vi "Build Rearange Frames by Index Array.vi"(9 "New Position":i32, 10 "Current Position":i32, 11 "N":i32) -> (2 "New Positions Array":i32[](array[numeric]))   [LabVIEW 2020]
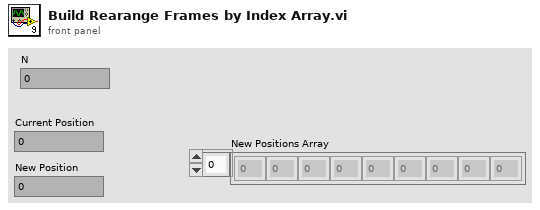
[diagram p1: front panel]
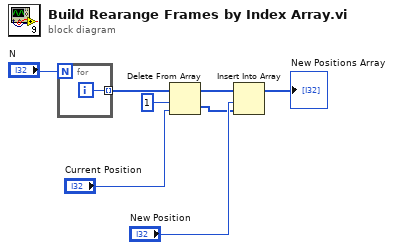
[diagram p0: block diagram]
diagram:
  n1 = for {
    N: "N" -> [_]
    tunnel: [w9] -> w4 mode=indexing
    i -> [w9]
  }
  n2 = Delete From Array(array=w4, length=1, index="Current Position") -> (deleted portion=w2:i32[], array with subset deleted=w1:i32[])
  n3 = Insert Into Array(array=w1, index="New Position", new element=w2) -> (→"New Positions Array":i32[])
